vi "ThrArray.vi"(8 "Error In":errorcluster, 10 "Threshold":dbl, 11 "Input Array":dbl[][](array[numeric])) -> (0 "Error Out":errorcluster, 3 "Array":dbl[][](array[numeric]))   [LabVIEW 2015]
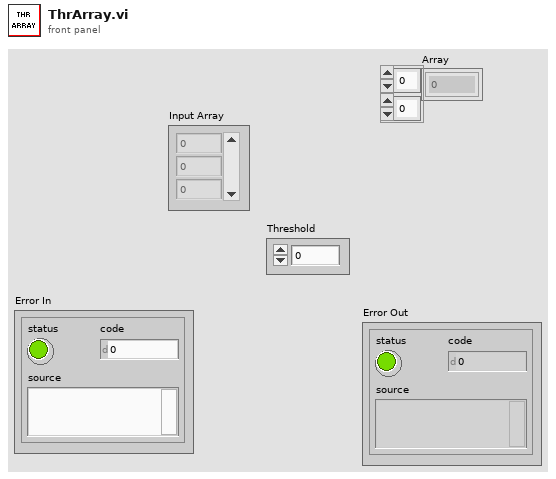
[diagram p1: front panel]
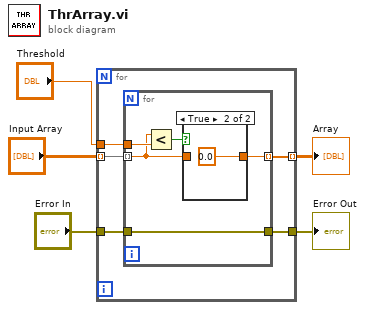
[diagram p0: block diagram]
diagram:
  n1 = for {
    tunnel: "Input Array" -> [w10] mode=indexing
    tunnel: "Threshold" -> [w9]
    tunnel: [w8] -> w3 mode=indexing
    tunnel: [w7] -> w2
    tunnel: "Error In" -> [w6]
    n2 = for {
      tunnel: [w14] -> w8 mode=indexing
      tunnel: w10 -> [w12] mode=indexing
      tunnel: w9 -> [w13]
      tunnel: [w11] -> w7
      tunnel: w6 -> [w11]
      n3 = Less?(x=w12, y=w13) -> (x < y?=w15:bool)
      n4 = case shown="True" w15 {
        tunnel: [w16 sgl 0.0] -> w14
        tunnel: w12 -> [w16 _]
        frame False {
        }
        frame True {
        }
      }
    }
  }
  "Array" <- w3
  "Error Out" <- w2
